vi "Load.vi"(8 "error in (no error)":errorcluster, 10 "JSON":string, 11 "Vision in":refnum<class "Vision.lvclass">) -> (0 "error out":errorcluster, 3 "Vision out":refnum<class "Vision.lvclass">)   [LabVIEW 2021, in "Vision.lvlib" / "Vision.lvclass"]
uses:
  Vision.lvclass
  Vision.lvclass/Vision.ctl
  <vilib>/userdefined/High Color/IMAQdx.ctl
  4fbf95c0-2566-4e16-a33f-654054b141f3.vi
  cf3bde78-90ca-47ba-b3a0-2da86aaaba43.vi
  <vilib>/JDP Science/JSONtext/String Subset.vi
  <vilib>/JDP Science/JSONtext/Parsing/Parse Full Path or Item Name.vi
  <vilib>/JDP Science/JSONtext/Next JSON Value.vi
  <vilib>/JDP Science/JSONtext/support/Error Cluster From Code.vi
  <vilib>/JDP Science/JSONtext/Offset/Find Item Locations by Path.vi
  <vilib>/JDP Science/JSONtext/JSON text to Variant.vi
  <vilib>/JDP Science/JSONtext/LVClass Serializer/JSONtext LVClass Serializer.lvclass
  <vilib>/JDP Science/JSONtext/JSONtext.lvlib
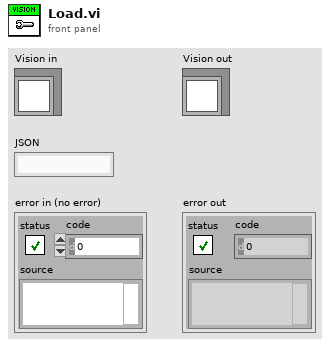
[diagram p1: front panel]
types:
  T1 = cluster{"Global Rectangle":i32[], "Contours":cluster{"Contour Type":u32, "ROI Type":u32, "Points":i32[]}[]}
  T2 = typedef "IMAQdx.ctl" = refnum<k21>
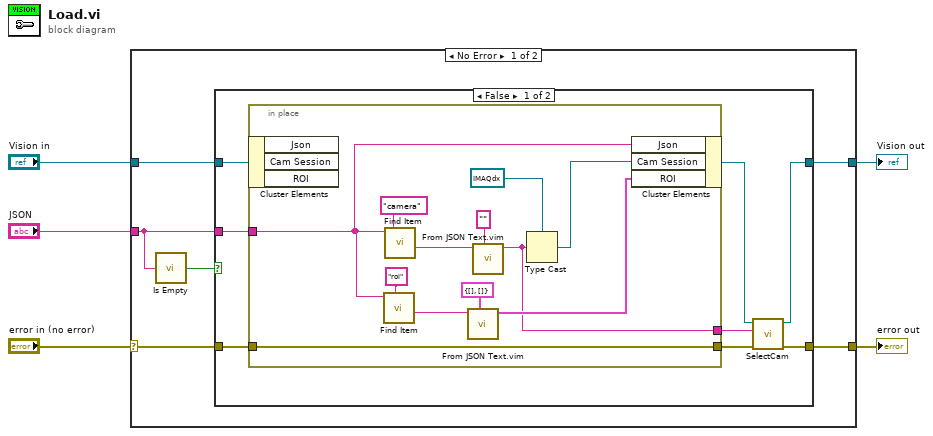
[diagram p0: block diagram]
diagram:
  n1 = case shown="No Error" "error in (no error)" {
    selector: "error in (no error)" -> [w10 w35]
    tunnel: [w6 w35] -> w4
    tunnel: [w7 w34] -> w2
    tunnel: "Vision in" -> [w11 w34]
    tunnel: "JSON" -> [w9 _]
    frame No Error {
      n2 = call <vilib>:"Is Empty.vi"("JSON"=w9) -> ("Empty"=w8:bool)  [unwired: 4 in]
      n3 = case shown="False" w8 {
        tunnel: w11 -> [w19 w33]
        tunnel: w10 -> [w18 w32]
        tunnel: w9 -> [w17 _]
        tunnel: [w14 w33] -> w7
        tunnel: [w13 w32] -> w6
        frame False {
          n4 = in-place {
            in-place-border: w18 -> [w27]
            in-place-border: w17 -> [w28]
            in-place-border: [w27] -> w16
            in-place-border: [w20] -> w12
            n5 = in-place-cluster #1(w19) -> ()  [unwired: 3 out]
            n6 = call <vilib>:"Find Item.vi"("$Path or Item Name"="roi", "JSON"=w28) -> ("<JSON>"=w26:string)  [unwired: 6 in, 3 out]
            n7 = call <vilib>:"Find Item.vi"("$Path or Item Name"="camera", "JSON"=w28) -> ("<JSON>"=w29:string)  [unwired: 6 in, 3 out]
            n8 = call "From JSON Text.vim"("Data Type and Default Value"=T1 {"Global Rectangle"=[], "Contours"=[]} ("ROI"), "JSON"=w26) -> ("Data out"=w24:T1)  [unwired: 8 in, 1 out]
            n9 = call "From JSON Text.vim"("Data Type and Default Value"="", "JSON"=w29) -> ("Data out"=w20:string)  [unwired: 8 in, 1 out]
            n10 = Type Cast(type=T2 refnum ("Cam Session"), x=w20) -> (*(type *) &x=w21:T2)
            n11 = in-place-cluster #1("Json"=w28, "Cam Session"=w21, "ROI"=w24) -> (w15:refnum<class "Vision.lvclass">)
          }
          n12 = call "SelectCam.vi"("error in (no error)"=w16, "Cam Session"=w12, "Vision in"=w15) -> ("error out"=w13:errorcluster, "Vision out"=w14:refnum<class "Vision.lvclass">)  [unwired: 7 in]
        }
        frame True {
        }
      }
    }
    frame Error {
    }
  }
  "error out" <- w4
  "Vision out" <- w2
